vi "CAENHV Get Bd Param Single.vi"(6 "slotList":u16[](array[numeric]), 7 "slotNum (1)":u16=1, 8 "error in (no error)":errorcluster, 9 "ParName":string, 11 "handle":i32) -> (0 "error out":errorcluster, 3 "ParValList":sgl[](array[numeric]))   [LabVIEW 2009, in "CAENHVWrapper.lvlib"]
doc: "CAENHVLIB_API CAENHVRESULT CAENHV_GetBdParam(int handle, \n ushort slotNum, const ushort *slotList, const char *ParName, void *ParValList);"
uses:
  <userlib>/CAENHVWrapper/CAENHVWrapper.lvlib
  <userlib>/CAENHVWrapper/CAENHVWrapper.dll
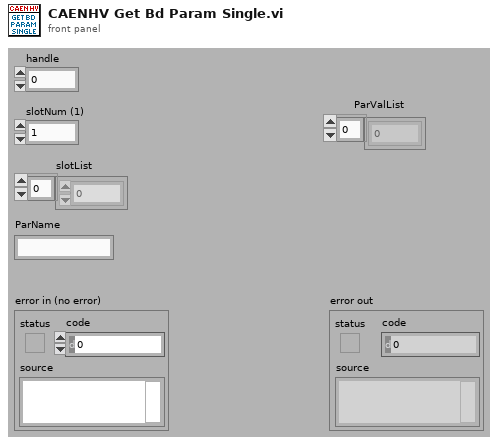
[diagram p1: front panel]
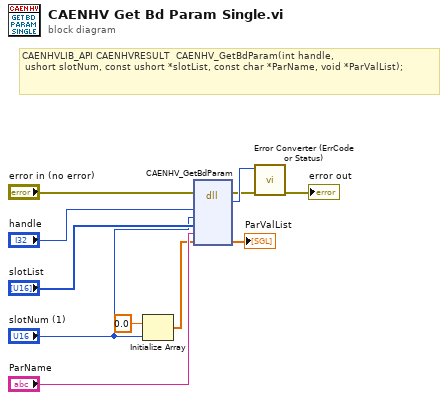
[diagram p0: block diagram]
diagram:
  # "CAENHVLIB_API CAENHVRESULT  CAENHV_GetBdParam(int handle, \n ushort slotNum, const ushort *slotList, const char *ParName, void *ParValList);"
  n1 = Initialize Array(sgl 0.0 ("ParValList"), "slotNum (1)") -> (w2:sgl[])
  n2 = dll-call lib="C:/Program Files/National Instruments/LabVIEW 2009/user.lib/CAENHVWrapper/CAENHVWrapper.*" fn="CAENHV_GetBdParam"(error in="error in (no error)", "handle"="handle", "slotNum"="slotNum (1)", "slotList"="slotList", "ParName"="ParName", "ParValList"=w2) -> (error out=w7:errorcluster, "return type"=w8:i32, "ParValList"=→"ParValList":sgl[])  [unwired: 6 in, 1 out]
  n3 = call <userlib>:"Error Converter (ErrCode or Status).vi"("error in (no error)"=w7, "error code"=w8) -> ("error out"=→"error out":errorcluster)  [unwired: 9 in]
